vi "Sequence.CreateStepLoop.vi"(7 "Iteration":string, 8 "error in (no error)":errorcluster, 10 "Duration":dbl, 11 "Elements":T1[](array[typedef])) -> (0 "error out":errorcluster, 3 "Tasks":refnum<k24>[](array[refnum]))   [LabVIEW 2013, in "Simple Sequence Tools - Editor.lvlib"]
uses:
  Simple Sequence Tools - Editor.lvlib
  NationalInstruments.VeriStand.RealTimeSequenceDefinitionApi
  Types/Compiled.StepElementProperties.ctl
  Shared/Types/ChannelProperties.ctl
  Shared/Types/StepTypes.ctl
  Shared/SubVIs/Constants.vi
  Shared/Simple Sequence Tools - Shared.lvlib
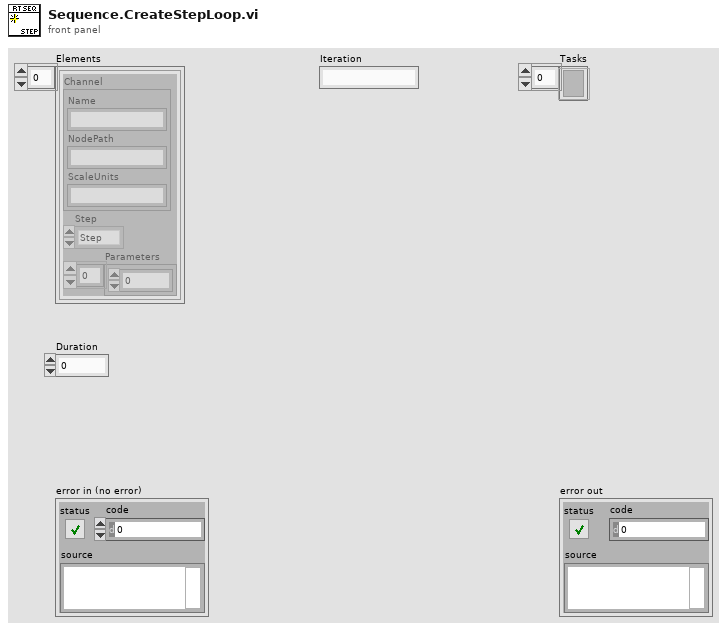
[diagram p1: front panel]
types:
  T1 = typedef "Simple Sequence Tools - Editor.lvlib/Compiled.StepElementProperties.ctl" = cluster{"Channel":T2, "Step":T3, "Parameters":dbl[]}
  T2 = typedef "Simple Sequence Tools - Shared.lvlib/ChannelProperties.ctl" = cluster{"Name":string, "NodePath":string, "ScaleUnits":string}
  T3 = typedef "Simple Sequence Tools - Shared.lvlib/StepTypes.ctl" = enum8{"Step", "iStep", "Ramp", "Unchanged", "Unknown"}
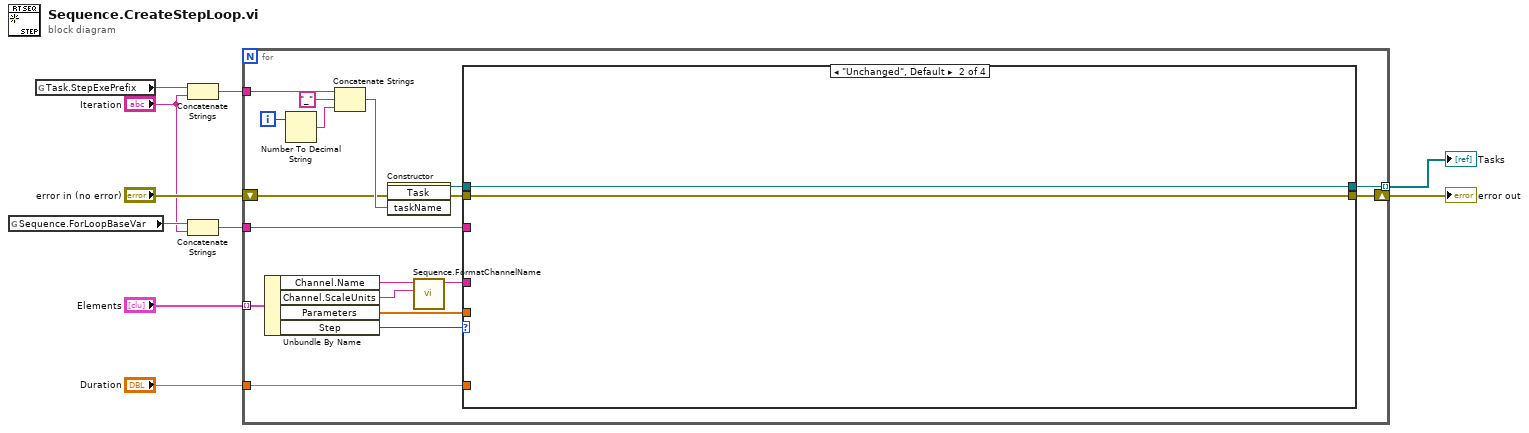
[diagram p0: block diagram]
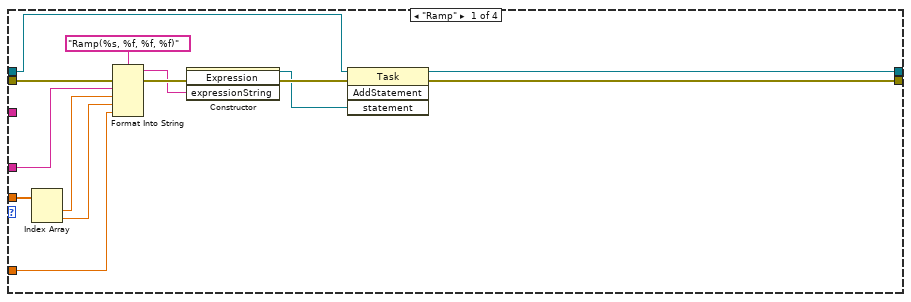
[diagram p2: hidden frame]
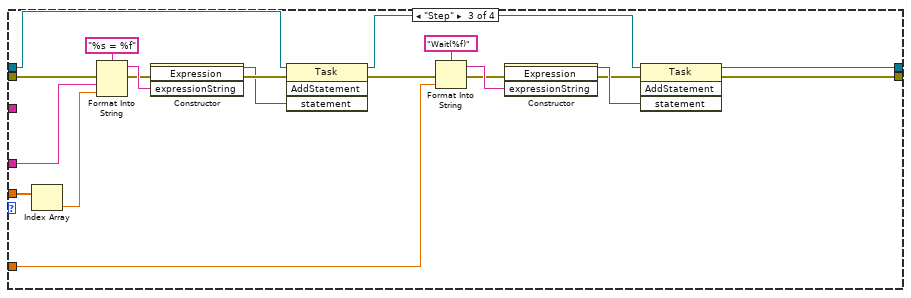
[diagram p3: hidden frame]
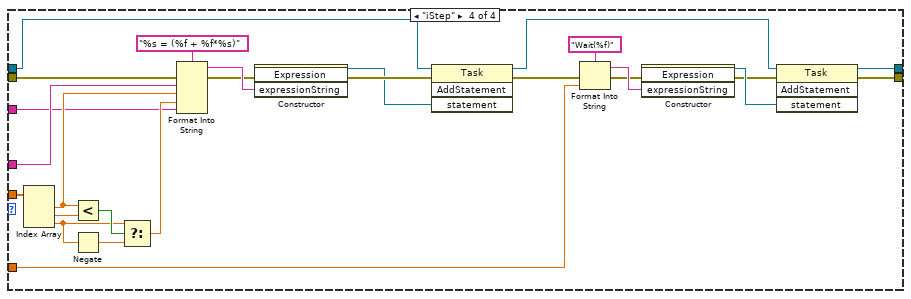
[diagram p4: hidden frame]
diagram:
  n1 = global read "Constants.vi" "Sequence.ForLoopBaseVar"() -> (w3:string)
  n2 = global read "Constants.vi" "Task.StepExePrefix"() -> (w5:string)
  n3 = Concatenate Strings(w5, "Iteration") -> (w4:string)
  n4 = Concatenate Strings(w3, "Iteration") -> (w1:string)
  n5 = for {
    tunnel: "Elements" -> [w23] mode=indexing
    shift-right: [w14] -> w9
    shift-left: "error in (no error)" -> [w22]
    tunnel: w4 -> [w27]
    tunnel: [w12] -> w10 mode=indexing
    tunnel: "Duration" -> [w18]
    tunnel: w1 -> [w11]
    i -> [w28]
    n6 = Unbundle By Name(w23) -> ("Channel.Name"=w21:string, "Channel.ScaleUnits"=w20:string, "Parameters"=w17:dbl[], "Step"=w16:T3)
    n7 = Number To Decimal String(number=w28) -> (decimal integer string=w25:string)  [unwired: 1 in]
    n8 = Concatenate Strings(w27, "_" ("string"), w25) -> (w24:string)
    n9 = constructor class="Task"(error in=w22, "taskName"=w24) -> (reference out=w13:refnum<k24>, error out=w15:errorcluster)  [unwired: 2 in, 2 out]
    n10 = call "Sequence.FormatChannelName.vi"("ScaleUnits"=w20, "Name"=w21) -> ("ChannelName"=w19:string)  [unwired: 9 in]
    n11 = case shown="\"Unchanged\", Default" w16 {
      tunnel: w19 -> [w41 _ w63 w89]
      tunnel: w17 -> [w40 _ w62 w88]
      tunnel: w18 -> [w37 _ w53 w80]
      tunnel: [w31 w43 w47 w74] -> w14
      tunnel: w15 -> [w36 w43 w60 w87]
      tunnel: w13 -> [w33 w44 w52 w79]
      tunnel: [w30 w44 w45 w72] -> w12
      tunnel: w11 -> [_ _ _ w65]
      frame "Ramp" {
        n12 = Index Array(array=w40) -> (element #1=w39:dbl, element #2=w38:dbl)  [unwired: 2 in]
        n13 = Format Into String(format string="Ramp(%s, %f, %f, %f)" ("expressionString"), error in=w36, w41, w39, w38, w37) -> (resulting string=w29:string, error out=w32:errorcluster)  [unwired: 1 in]
        n14 = constructor class="Expression"(error in=w32, "expressionString"=w29) -> (reference out=w34:refnum<k24>, error out=w35:errorcluster)  [unwired: 2 in, 2 out]
        n15 = invoke class="Task" method="AddStatement"(reference=w33, error in=w35, "statement"=w34) -> (reference out=w30:refnum<k24>, error out=w31:errorcluster)  [unwired: 1 in, 2 out]
      }
      frame "Unchanged", Default {
      }
      frame "Step" {
        n16 = Index Array(array=w62) -> (element=w61:dbl)  [unwired: 1 in]
        n17 = Format Into String(format string="%s = %f" ("expressionString"), error in=w60, w63, w61) -> (resulting string=w57:string, error out=w48:errorcluster)  [unwired: 1 in]
        n18 = constructor class="Expression"(error in=w48, "expressionString"=w57) -> (reference out=w58:refnum<k24>, error out=w59:errorcluster)  [unwired: 2 in, 2 out]
        n19 = invoke class="Task" method="AddStatement"(reference=w52, error in=w59, "statement"=w58) -> (reference out=w46:refnum<k24>, error out=w49:errorcluster)  [unwired: 1 in, 2 out]
        n20 = Format Into String(format string="Wait(%f)", error in=w49, w53) -> (resulting string=w51:string, error out=w50:errorcluster)  [unwired: 1 in]
        n21 = constructor class="Expression"(error in=w50, "expressionString"=w51) -> (reference out=w56:refnum<k24>, error out=w55:errorcluster)  [unwired: 2 in, 2 out]
        n22 = invoke class="Task" method="AddStatement"(reference=w46, error in=w55, "statement"=w56) -> (reference out=w45:refnum<k24>, error out=w47:errorcluster)  [unwired: 1 in, 2 out]
      }
      frame "iStep" {
        n23 = Index Array(array=w88) -> (element #1=w71:dbl, element #2=w70:dbl, element #3=w67:dbl)  [unwired: 3 in]
        n24 = Less?(x=w71, y=w70) -> (x < y?=w69:bool)
        n25 = Negate(x=w67) -> (-x=w68:dbl)
        n26 = Select(t=w67, s=w69, f=w68) -> (s? t:f=w66:dbl)
        n27 = Format Into String(format string="%s = (%f + %f*%s)" ("expressionString"), error in=w87, w89, w71, w66, w65) -> (resulting string=w84:string, error out=w75:errorcluster)  [unwired: 1 in]
        n28 = constructor class="Expression"(error in=w75, "expressionString"=w84) -> (reference out=w85:refnum<k24>, error out=w86:errorcluster)  [unwired: 2 in, 2 out]
        n29 = invoke class="Task" method="AddStatement"(reference=w79, error in=w86, "statement"=w85) -> (reference out=w73:refnum<k24>, error out=w76:errorcluster)  [unwired: 1 in, 2 out]
        n30 = Format Into String(format string="Wait(%f)", error in=w76, w80) -> (resulting string=w78:string, error out=w77:errorcluster)  [unwired: 1 in]
        n31 = constructor class="Expression"(error in=w77, "expressionString"=w78) -> (reference out=w83:refnum<k24>, error out=w82:errorcluster)  [unwired: 2 in, 2 out]
        n32 = invoke class="Task" method="AddStatement"(reference=w73, error in=w82, "statement"=w83) -> (reference out=w72:refnum<k24>, error out=w74:errorcluster)  [unwired: 1 in, 2 out]
      }
    }
  }
  "Tasks" <- w10
  "error out" <- w9
